vi "GENser Checksum Verify.vi"(8 "error":errorcluster, 10 "String in":string, 11 "VISA":refnum<visa-resource-name>="COM1") -> (0 "error out":errorcluster, 2 "Trimmed String":string, 3 "VISA out":refnum<visa-resource-name>)   [LabVIEW 2017]
doc: "This vi will verify the checksum at the end of the response message from the Genesys power supply. The checksum format is: \n \"String\" & \"Dollar Sign\" & \"Checksum with Two Hex Digits\"\n\nIf a checksum error is detected, the error will be shown in the \"error out\" cluster. \nThe \"Trimmed String\" is \"String in\" minus the checksum and terminators"
panel:
  # "Verify Checksum"
  # "Lambda Genesys \n Serial Port\n  DC Power Supplies"
  # "Verify the  \"$xx\" checksum which\nwas appended to end of any \nresponse string"
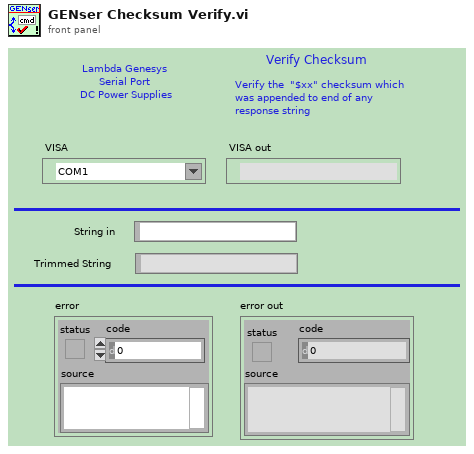
[diagram p1: front panel]
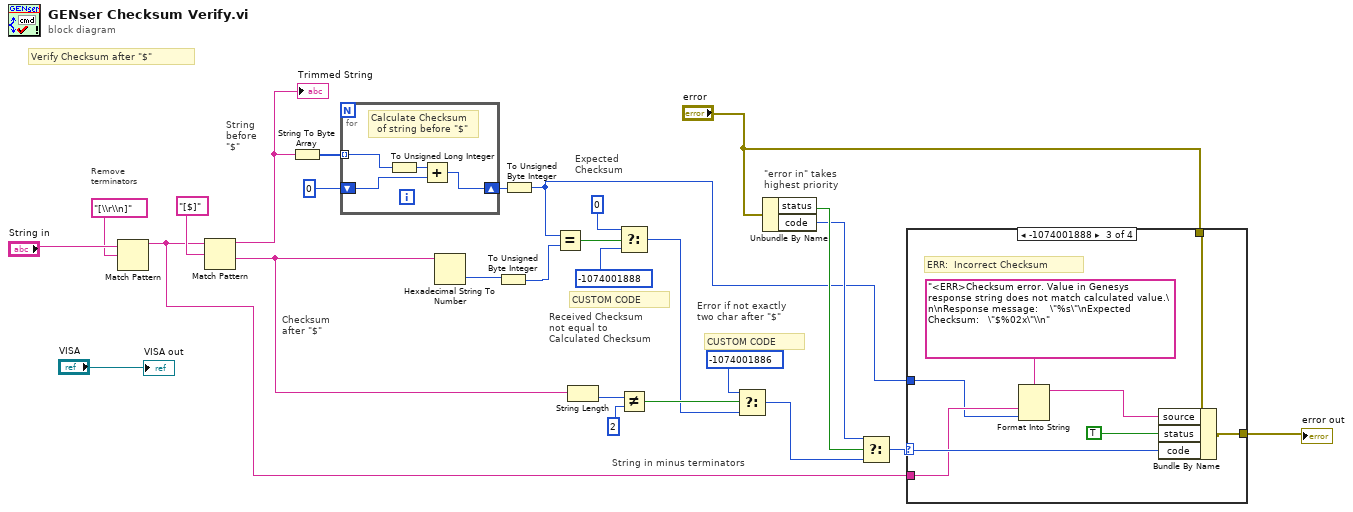
[diagram p0: block diagram]
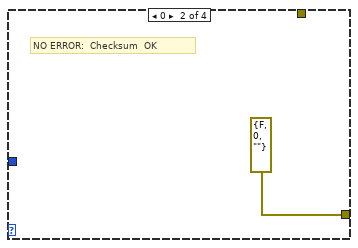
[diagram p3: hidden frame]
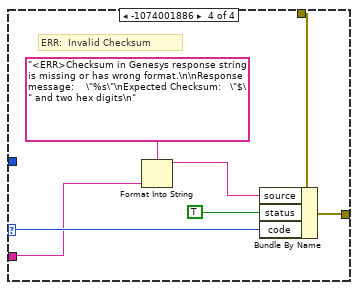
[diagram p4: hidden frame]
diagram:
  # "Expected\nChecksum"
  # "String in minus terminators"
  # "\"error in\" takes\nhighest priority"
  # "String\nbefore\n\"$\""
  # "Checksum\nafter \"$\""
  # "CUSTOM CODE"
  # "Received Checksum\nnot equal to\nCalculated Checksum"
  # "Error if not exactly\ntwo char after \"$\""
  # "CUSTOM CODE"
  # "Remove\nterminators"
  # "Verify Checksum after \"$\""
  n1 = Match Pattern(string="String in", regular expression="[\\r\\n]") -> (before substring=w3:string)  [unwired: 1 in, 3 out]
  n2 = Match Pattern(string=w3, regular expression="[$]") -> (before substring=w4:string, after substring=w17:string)  [unwired: 1 in, 2 out]
  "Trimmed String" <- w4
  n3 = String To Byte Array(string=w4) -> (unsigned byte array=w24:u8[])
  n4 = for {
    tunnel: w24 -> [w31] mode=indexing
    shift-right: [w29] -> w2
    shift-left: u32 0 -> [w30]
    # "Calculate Checksum\n  of string before \"$\""
    n5 = To Unsigned Long Integer(number=w31) -> (unsigned 32bit integer=w28:u32)
    n6 = Add(x=w28, y=w30) -> (x+y=w29:u32)
  }
  n7 = Hexadecimal String To Number(string=w17) -> (number=w16:u32)  [unwired: 2 in, 1 out]
  n8 = To Unsigned Byte Integer(number=w16) -> (unsigned 8bit integer=w15:u8)
  n9 = To Unsigned Byte Integer(number=w2) -> (unsigned 8bit integer=w1:u8)
  n10 = Equal?(x=w1, y=w15) -> (x = y?=w14:bool)
  n11 = String Length(string=w17) -> (length=w21:i32)
  n12 = Select(t=0 ("code"), s=w14, f=-1074001888 ("code")) -> (s? t:f=w12:i32)
  n13 = Not Equal?(x=w21, y=2) -> (x != y?=w19:bool)
  n14 = Select(t=-1074001886 ("code"), s=w19, f=w12) -> (s? t:f=w6:i32)
  n15 = Unbundle By Name("error") -> ("status"=w8:bool, "code"=w7:i32)
  n16 = Select(t=w7, s=w8, f=w6) -> (s? t:f=w5:i32)
  n17 = case shown="-1074001888" w5 {
    selector: w5 -> [_ _ w39 w45]
    tunnel: "error" -> [w32 _ w40 w47]
    tunnel: [w32 errorcluster {"status"=FALSE, "code"=0, "source"=""} ("error IO") w36 w46] -> w10
    tunnel: w3 -> [_ _ w38 w42]
    tunnel: w1 -> [_ _ w37 _]
    frame -1, Default {
      # "ERR:  Generic VISA"
    }
    frame 0 {
      # "NO ERROR:  Checksum  OK"
    }
    frame -1074001888 {
      # "ERR:  Incorrect Checksum"
      n18 = Format Into String(format string="<ERR>Checksum error. Value in Genesys response string does not match calculated value.\n\nResponse message:    \"%s\"\nExpected Checksum:   \"$%02x\"\\n" ("Source (VI Name)"), w38, w37) -> (resulting string=w35:string)  [unwired: 2 in, 1 out]
      n19 = Bundle By Name(cluster=w40, "source"=w35, "status"=TRUE, "code"=w39) -> (w36:errorcluster)
    }
    frame -1074001886 {
      # "ERR:  Invalid Checksum"
      n20 = Format Into String(format string="<ERR>Checksum in Genesys response string is missing or has wrong format.\n\nResponse message:    \"%s\"\nExpected Checksum:   \"$\" and two hex digits\n" ("Source (VI Name)"), w42) -> (resulting string=w43:string)  [unwired: 2 in, 1 out]
      n21 = Bundle By Name(cluster=w47, "source"=w43, "status"=TRUE, "code"=w45) -> (w46:errorcluster)
    }
  }
  "error out" <- w10
  "VISA out" <- "VISA"
